vi "CRYAlign Steps VI Center.vi"(8 "Tab2":refnum<vi>, 9 "Tab1":refnum<vi>, 10 "Input/Output":bool, 11 "VIRef":refnum<vi>) -> ()   [LabVIEW 2013]
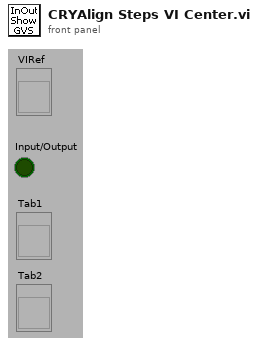
[diagram p1: front panel]
types:
  T1 = enum16{"Always On", "Always Off", "Off While Running"}
  T2 = typedef "LVPointTypeDef.ctl" = cluster{"Horizontal":i16, "Vertical":i16}
  T3 = typedef "LVBoundsTypeDef.ctl" = cluster{"Width":u32, "Height":u32}
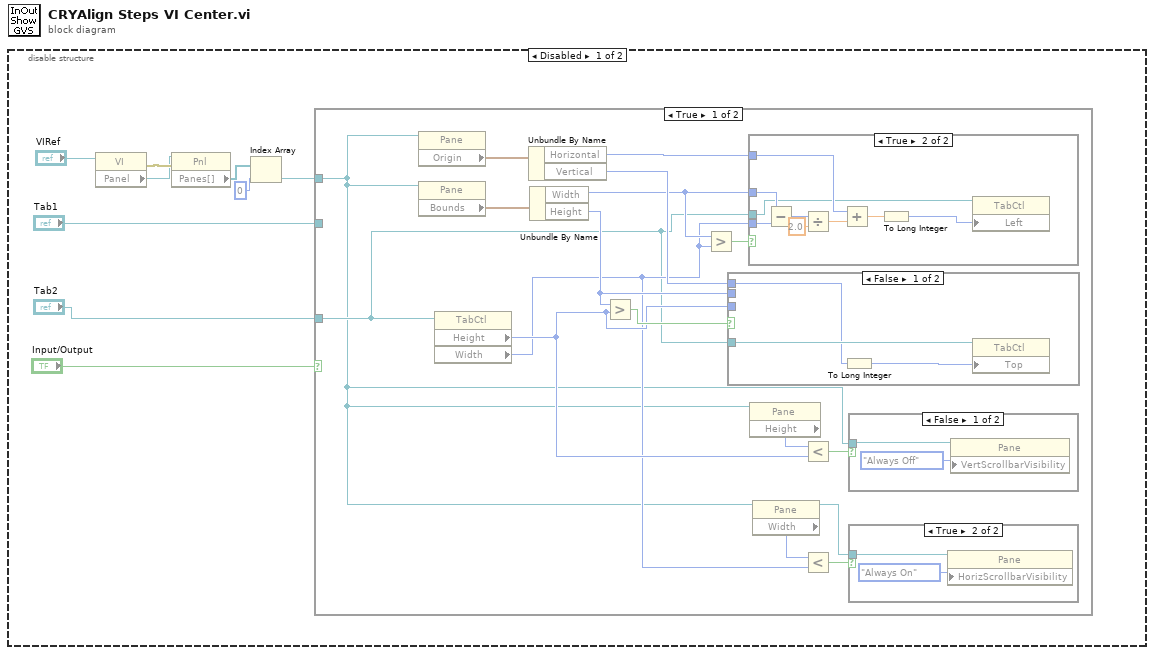
[diagram p0: block diagram]
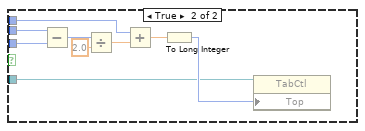
[diagram p2: hidden frame]
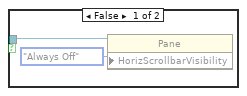
[diagram p3: hidden frame]
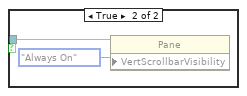
[diagram p4: hidden frame]
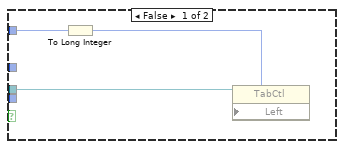
[diagram p5: hidden frame]
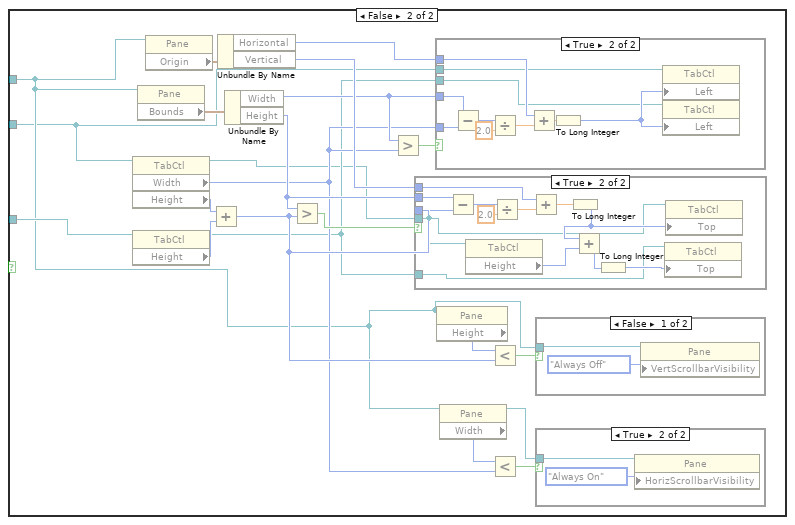
[diagram p6: hidden frame]
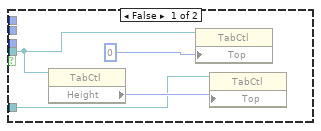
[diagram p7: hidden frame]
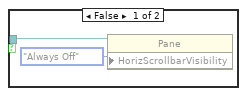
[diagram p8: hidden frame]
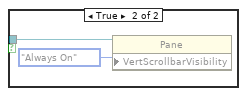
[diagram p9: hidden frame]
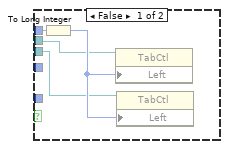
[diagram p10: hidden frame]
diagram:
  n1 = disable-structure shown="Disabled" {
    frame Disabled {
      n2 = property class="VI"(reference="VIRef") -> (error out=w6:errorcluster, "Panel"=w1:refnum<vi>)  [unwired: 1 in, 1 out]
      n3 = property class="Pnl"(reference=w1, error in=w6) -> ("Panes[]"=w5:refnum<vi>[])  [unwired: 2 out]
      n4 = Index Array(array=w5, index=0) -> (element=w2:refnum<vi>)
      n5 = case shown="True" "Input/Output" {
        tunnel: w2 -> [w10 w62]
        tunnel: "Tab1" -> [_ w59]
        tunnel: "Tab2" -> [w11 w63]
        frame True {
          n6 = property class="Pane"(reference=w10) -> ("Origin"=w17:T2)  [unwired: 1 in, 2 out]
          n7 = property class="Pane"(reference=w10) -> ("Bounds"=w16:T3)  [unwired: 1 in, 2 out]
          n8 = property on="Property Node" class="TabCtl"(reference=w11) -> ("Height"=w13:u32, "Width"=w12:u32)  [unwired: 1 in, 2 out]
          n9 = Unbundle By Name(w17) -> ("Horizontal"=w25:i16, "Vertical"=w18:i16)
          n10 = Unbundle By Name(w16) -> ("Width"=w14:u32, "Height"=w15:u32)
          n11 = Greater?(x=w15, y=w13) -> (0:w19:bool)
          n12 = Greater?(x=w14, y=w12) -> (0:w26:bool)
          n13 = case shown="False" w19 {
            tunnel: w15 -> [_ w36]
            tunnel: w13 -> [_ w35]
            tunnel: w18 -> [w28 w32]
            tunnel: w11 -> [w29 w30]
            frame False {
              n14 = To Long Integer(number=w28) -> (32bit integer=w27:i32)
              n15 = property on="Property Node" class="TabCtl"(reference=w29, "Top"=w27) -> ()  [unwired: 1 in, 2 out]
            }
            frame True {
              n16 = Subtract(x=w36, y=w35) -> (x-y=w38:u32)
              n17 = Divide(x=w38, y=2.0) -> (x/y=w33:dbl)
              n18 = Add(x=w32, y=w33) -> (x+y=w34:dbl)
              n19 = To Long Integer(number=w34) -> (32bit integer=w31:i32)
              n20 = property on="Property Node" class="TabCtl"(reference=w30, "Top"=w31) -> ()  [unwired: 1 in, 2 out]
            }
          }
          n21 = case shown="True" w26 {
            tunnel: w12 -> [_ w58]
            tunnel: w25 -> [w49 w54]
            tunnel: w14 -> [_ w57]
            tunnel: w11 -> [w47 w50]
            frame False {
              n22 = To Long Integer(number=w49) -> (32bit integer=w48:i32)
              n23 = property on="Property Node" class="TabCtl"(reference=w47, "Left"=w48) -> ()  [unwired: 1 in, 2 out]
            }
            frame True {
              n24 = Subtract(x=w57, y=w58) -> (x-y=w55:u32)
              n25 = Divide(x=w55, y=2.0) -> (x/y=w53:dbl)
              n26 = Add(x=w54, y=w53) -> (x+y=w52:dbl)
              n27 = To Long Integer(number=w52) -> (32bit integer=w51:i32)
              n28 = property on="Property Node" class="TabCtl"(reference=w50, "Left"=w51) -> ()  [unwired: 1 in, 2 out]
            }
          }
          n29 = property class="Pane"(reference=w10) -> ("Height"=w20:u32)  [unwired: 1 in, 2 out]
          n30 = property class="Pane"(reference=w10) -> (reference out=w24:refnum<vi>, "Width"=w23:u32)  [unwired: 1 in, 1 out]
          n31 = Less?(x=w20, y=w13) -> (x < y?=w21:bool)
          n32 = Less?(x=w23, y=w12) -> (x < y?=w22:bool)
          n33 = case shown="False" w21 {
            tunnel: w10 -> [w43 w45]
            frame False {
              n34 = property class="Pane"(reference=w43, "VertScrollbarVisibility"=T1."Always Off" ("Horizontal Scrollbar Visibility")) -> ()  [unwired: 1 in, 2 out]
            }
            frame True {
              n35 = property class="Pane"(reference=w45, "VertScrollbarVisibility"=T1."Always On" ("Horizontal Scrollbar Visibility")) -> ()  [unwired: 1 in, 2 out]
            }
          }
          n36 = case shown="True" w22 {
            tunnel: w24 -> [w39 w41]
            frame False {
              n37 = property class="Pane"(reference=w39, "HorizScrollbarVisibility"=T1."Always Off" ("Horizontal Scrollbar Visibility")) -> ()  [unwired: 1 in, 2 out]
            }
            frame True {
              n38 = property class="Pane"(reference=w41, "HorizScrollbarVisibility"=T1."Always On" ("Horizontal Scrollbar Visibility")) -> ()  [unwired: 1 in, 2 out]
            }
          }
        }
        frame False {
          n39 = property on="Property Node" class="TabCtl"(reference=w59) -> (reference out=w60:refnum<vi>, "Width"=w64:u32, "Height"=w73:u32)  [unwired: 1 in, 1 out]
          n40 = property on="Property Node" class="TabCtl"(reference=w63) -> (reference out=w61:refnum<vi>, "Height"=w72:u32)  [unwired: 1 in, 1 out]
          n41 = property class="Pane"(reference=w62) -> ("Bounds"=w68:T3)  [unwired: 1 in, 2 out]
          n42 = property class="Pane"(reference=w62) -> ("Origin"=w69:T2)  [unwired: 1 in, 2 out]
          n43 = Add(x=w73, y=w72) -> (x+y=w65:u32)
          n44 = Unbundle By Name(w69) -> ("Horizontal"=w79:i16, "Vertical"=w70:i16)
          n45 = Unbundle By Name(w68) -> ("Width"=w66:u32, "Height"=w67:u32)
          n46 = Greater?(x=w67, y=w65) -> (0:w71:bool)
          n47 = Greater?(x=w66, y=w64) -> (0:w80:bool)
          n48 = case shown="True" w71 {
            tunnel: w67 -> [_ w95]
            tunnel: w65 -> [_ w94]
            tunnel: w70 -> [_ w91]
            tunnel: w61 -> [w82 w85]
            tunnel: w60 -> [w81 w86]
            frame False {
              n49 = property on="Property Node" class="TabCtl"(reference=w81) -> ("Height"=w83:u32)  [unwired: 1 in, 2 out]
              n50 = property on="Property Node" class="TabCtl"(reference=w81, "Top"=0 ("Position:Top")) -> ()  [unwired: 1 in, 2 out]
              n51 = property on="Property Node" class="TabCtl"(reference=w82, "Top"=w83) -> ()  [unwired: 1 in, 2 out]
            }
            frame True {
              n52 = Subtract(x=w95, y=w94) -> (x-y=w97:u32)
              n53 = property on="Property Node" class="TabCtl"(reference=w86) -> ("Height"=w88:u32)  [unwired: 1 in, 2 out]
              n54 = Divide(x=w97, y=2.0) -> (x/y=w92:dbl)
              n55 = Add(x=w91, y=w92) -> (x+y=w93:dbl)
              n56 = To Long Integer(number=w93) -> (32bit integer=w89:i32)
              n57 = Add(x=w89, y=w88) -> (x+y=w90:u32)
              n58 = To Long Integer(number=w90) -> (32bit integer=w87:i32)
              n59 = property on="Property Node" class="TabCtl"(reference=w85, "Top"=w87) -> ()  [unwired: 1 in, 2 out]
              n60 = property on="Property Node" class="TabCtl"(reference=w86, "Top"=w89) -> ()  [unwired: 1 in, 2 out]
            }
          }
          n61 = case shown="True" w80 {
            tunnel: w64 -> [_ w119]
            tunnel: w79 -> [w109 w115]
            tunnel: w66 -> [_ w118]
            tunnel: w59 -> [w107 w111]
            tunnel: w61 -> [w106 w110]
            frame False {
              n62 = To Long Integer(number=w109) -> (32bit integer=w108:i32)
              n63 = property on="Property Node" class="TabCtl"(reference=w107, "Left"=w108) -> ()  [unwired: 1 in, 2 out]
              n64 = property on="Property Node" class="TabCtl"(reference=w106, "Left"=w108) -> ()  [unwired: 1 in, 2 out]
            }
            frame True {
              n65 = Subtract(x=w118, y=w119) -> (x-y=w116:u32)
              n66 = Divide(x=w116, y=2.0) -> (x/y=w114:dbl)
              n67 = Add(x=w115, y=w114) -> (x+y=w113:dbl)
              n68 = To Long Integer(number=w113) -> (32bit integer=w112:i32)
              n69 = property on="Property Node" class="TabCtl"(reference=w111, "Left"=w112) -> ()  [unwired: 1 in, 2 out]
              n70 = property on="Property Node" class="TabCtl"(reference=w110, "Left"=w112) -> ()  [unwired: 1 in, 2 out]
            }
          }
          n71 = property class="Pane"(reference=w62) -> ("Height"=w74:u32)  [unwired: 1 in, 2 out]
          n72 = property class="Pane"(reference=w62) -> (reference out=w78:refnum<vi>, "Width"=w77:u32)  [unwired: 1 in, 1 out]
          n73 = Less?(x=w74, y=w65) -> (x < y?=w75:bool)
          n74 = Less?(x=w77, y=w64) -> (x < y?=w76:bool)
          n75 = case shown="False" w75 {
            tunnel: w62 -> [w102 w104]
            frame False {
              n76 = property class="Pane"(reference=w102, "VertScrollbarVisibility"=T1."Always Off" ("Horizontal Scrollbar Visibility")) -> ()  [unwired: 1 in, 2 out]
            }
            frame True {
              n77 = property class="Pane"(reference=w104, "VertScrollbarVisibility"=T1."Always On" ("Horizontal Scrollbar Visibility")) -> ()  [unwired: 1 in, 2 out]
            }
          }
          n78 = case shown="True" w76 {
            tunnel: w78 -> [w98 w100]
            frame False {
              n79 = property class="Pane"(reference=w98, "HorizScrollbarVisibility"=T1."Always Off" ("Horizontal Scrollbar Visibility")) -> ()  [unwired: 1 in, 2 out]
            }
            frame True {
              n80 = property class="Pane"(reference=w100, "HorizScrollbarVisibility"=T1."Always On" ("Horizontal Scrollbar Visibility")) -> ()  [unwired: 1 in, 2 out]
            }
          }
        }
      }
    }
    frame Enabled {
    }
  }
